vi "Define Encryption.vi"(8 "error in (no error)":errorcluster, 10 "Encryption Method":refnum<class "Encryption.lvclass">, 11 "Log in":refnum<class "Log.lvclass">) -> (0 "error out":errorcluster, 3 "Log out":refnum<class "Log.lvclass">)   [LabVIEW 2019, in "TSC Event Logger.lvlib" / "Log.lvclass"]
doc: "Define an encryption method for the project.\n\n<b>Code Developed By:</b>\nTechnology Service Corporation\nBloomington, IN 47403\nwww.tsc.com/atcs\n\nDeveloper:\nDaniel Coons"
uses:
  Log.lvclass
  Encryption/Encryption.lvclass
  Log.lvclass/Log.ctl
  Log Sinks/Log Sinks.lvclass/Log Sinks.ctl
  Log Sinks/Log Sinks.lvclass
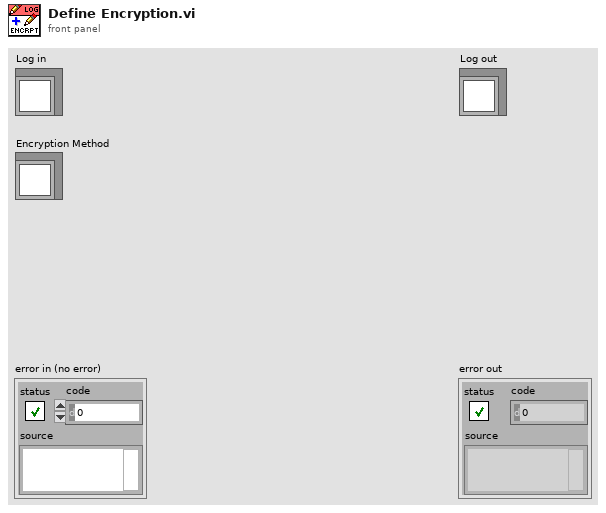
[diagram p1: front panel]
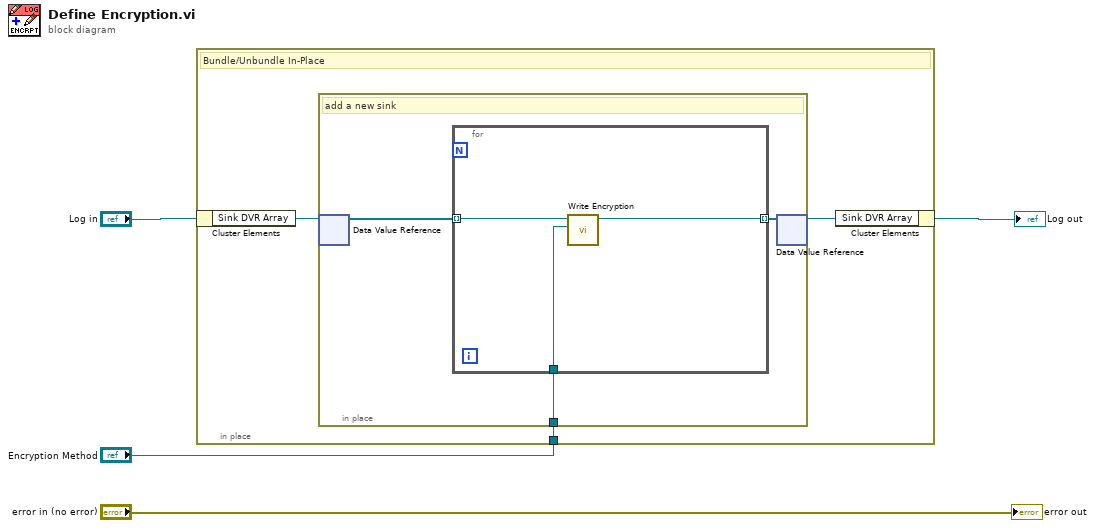
[diagram p0: block diagram]
diagram:
  n1 = in-place {
    in-place-border: "Encryption Method" -> [w5]
    # "Bundle/Unbundle In-Place"
    n2 = in-place-cluster #1("Log in") -> ("Sink DVR Array"=w7:refnum<data-value>)
    n3 = in-place {
      in-place-border: w5 -> [w8]
      # "add a new sink"
      n4 = in-place-dvr #2(w7) -> (w10:refnum<class "Log Sinks.lvclass">[])  [unwired: 1 out]
      n5 = for {
        tunnel: w10 -> [w11] mode=indexing
        tunnel: [w13] -> w9 mode=indexing
        tunnel: w8 -> [w12]
        n6 = call "Write Encryption.vi"("TSC Event Logger.lvlib:Encryption.lvclass"=w12, "Log Sinks in"=w11) -> ("Log Sinks out"=w13:refnum<class "Log Sinks.lvclass">)  [unwired: 8 in, 1 out]
      }
      n7 = in-place-dvr #2(w9) -> (w6:refnum<data-value>)  [unwired: 1 out]
    }
    n8 = in-place-cluster #1("Sink DVR Array"=w6) -> (→"Log out":refnum<class "Log.lvclass">)
  }
  "error out" <- "error in (no error)"
